vi "FPGA Wizard.vi"() -> ()   [LabVIEW 2015]
uses:
  Classes/Project/FPGA Settings.ctl
  Classes/Module/Module Class/Module Settings.ctl
  Classes/IO/IO Class/Signal Settings.ctl
  Classes/Project/Project.lvclass
  Classes/Loop/Block Diagram/Block Diagram.lvclass
  Classes/IO/IO Class/IO Class.lvclass
  Classes/Module/Module Class/Module.lvclass
panel:
  out "Array":T1[](array[typedef])
  out "error out":errorcluster
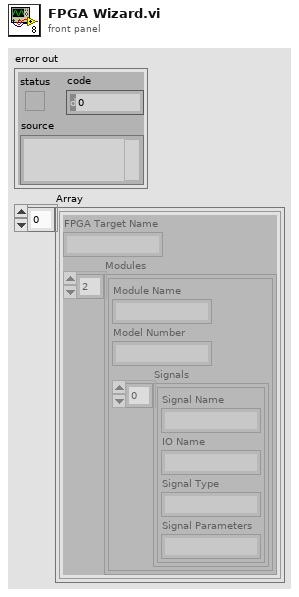
[diagram p1: front panel]
types:
  T1 = typedef "FPGA Settings.ctl" = cluster{"FPGA Target Name":string, "Modules":T2[]}
  T2 = typedef "Module.lvclass/Module Settings.ctl" = cluster{"Module Name":string, "Model Number":string, "Signals":T3[]}
  T3 = typedef "IO Class.lvclass/Signal Settings.ctl" = cluster{"Signal Name":string, "IO Name":string, "Signal Type":string, "Signal Parameters":string}
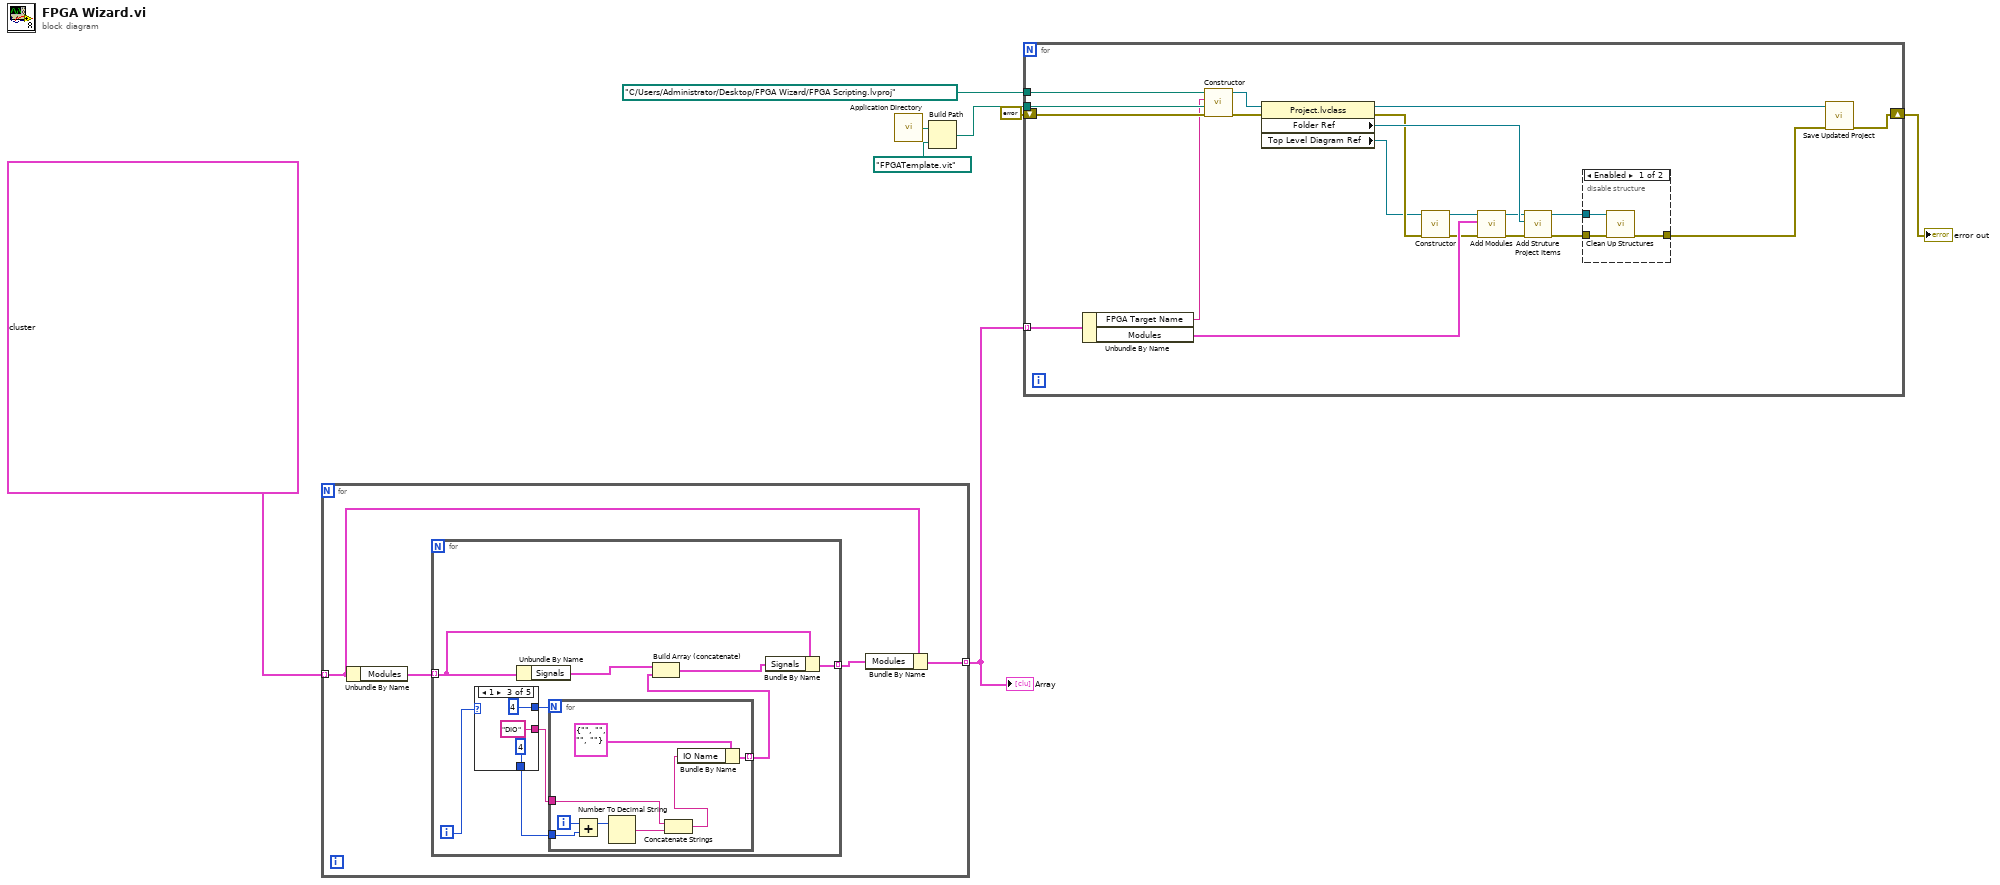
[diagram p0: block diagram]
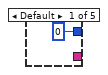
[diagram p2: hidden frame]
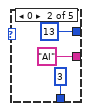
[diagram p3: hidden frame]
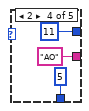
[diagram p4: hidden frame]
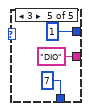
[diagram p5: hidden frame]
diagram:
  n1 = for {
    tunnel: T1[] [{"FPGA Target Name"="FPGA Target", "Modules"=[{"Module Name"="Mod1", "Model Number"="9220", "Signals"=[{"Signal Name"="Press", "IO Name"="AI0", "Signal Type"="Numeric Indicator", "Signal Parameters"=""}, {"Signal Name"="Temp", "IO Name"="AI1", "Signal Type"="Numeric Indicator", "Signal Parameters"=""}, {"Signal Name"="Injector", "IO Name"="AI2", "Signal Type"="Analog PWM Input", "Signal Parameters"=""}]}, {"Module Name"="Mod2", "Model Number"="9401", "Signals"=[{"Signal Name"="Relay State", "IO Name"="DIO0", "Signal Type"="Digital Indicator", "Signal Parameters"=""}, {"Signal Name"="Switch State", "IO Name"="DIO1", "Signal Type"="Digital Indicator", "Signal Parameters"=""}, {"Signal Name"="Key State", "IO Name"="DIO2", "Signal Type"="Digital Static Input", "Signal Parameters"=""}, {"Signal Name"="PWM State", "IO Name"="DIO3", "Signal Type"="Digital PWM Input", "Signal Parameters"=""}, {"Signal Name"="Cylinder 1 Injector", "IO Name"="DIO3", "Signal Type"="Digital Event", "Signal Parameters"="{\"Events\":4}"}]}, {"Module Name"="Mod3", "Model Number"="9264", "Signals"=[{"Signal Name"="Dyno Setpoint", "IO Name"="AO0", "Signal Type"="Numeric Control", "Signal Parameters"=""}, {"Signal Name"="Power Supply Setpoint", "IO Name"="AO1", "Signal Type"="Numeric Control", "Signal Parameters"=""}, {"Signal Name"="VR Sensor", "IO Name"="AO3", "Signal Type"="Analog Replay", "Signal Parameters"=""}, {"Signal Name"="Knock", "IO Name"="AO3", "Signal Type"="Knock Sensor", "Signal Parameters"="{\"Cyclinders\":6}"}, {"Signal Name"="Simple Knock", "IO Name"="AO4", "Signal Type"="Sine Output", "Signal Parameters"=""}]}, {"Module Name"="Mod4", "Model Number"="9401", "Signals"=[{"Signal Name"="Intake CAM", "IO Name"="DIO0", "Signal Type"="Digital Pattern", "Signal Parameters"=""}, {"Signal Name"="Exhaust CAM", "IO Name"="DIO1", "Signal Type"="Digital Pattern", "Signal Parameters"=""}, {"Signal Name"="Crank", "IO Name"="DIO2", "Signal Type"="Directional Sensor", "Signal Parameters"=""}, {"Signal Name"="Relay", "IO Name"="DIO3", "Signal Type"="Digital Control", "Signal Parameters"=""}, {"Signal Name"="Switch", "IO Name"="DIO4", "Signal Type"="Digital Control", "Signal Parameters"=""}, {"Signal Name"="PWM", "IO Name"="DIO5", "Signal Type"="Digital PWM Output", "Signal Parameters"=""}, {"Signal Name"="Key", "IO Name"="DIO6", "Signal Type"="Digital Static Output", "Signal Parameters"=""}]}, {"Module Name"="Mod5", "Model Number"="9401", "Signals"=[{"Signal Name"="Front Driver Wheel Speed", "IO Name"="DIO0, DIO1", "Signal Type"="Wheel Speed Sensor", "Signal Parameters"=""}, {"Signal Name"="Front Passenger Wheel Speed", "IO Name"="DIO2, DIO3", "Signal Type"="Wheel Speed Sensor", "Signal Parameters"=""}, {"Signal Name"="Rear Driver Wheel Speed", "IO Name"="DIO4, DIO5", "Signal Type"="Wheel Speed Sensor", "Signal Parameters"=""}, {"Signal Name"="Rear Passenger Wheel Speed", "IO Name"="DIO6,DIO7", "Signal Type"="Wheel Speed Sensor", "Signal Parameters"=""}]}]}] -> [w11] mode=indexing
    tunnel: [w9] -> w1 mode=indexing
    n2 = Unbundle By Name(w11) -> ("Modules"=w12:T2[])
    n3 = for {
      tunnel: w12 -> [w18] mode=indexing
      tunnel: [w16] -> w10 mode=indexing
      i -> [w15]
      n4 = case shown="1" w15 {
        tunnel: [0 13 4 11 1] -> w21
        tunnel: [_ "AI" "DIO" "AO" "DIO"] -> w14
        tunnel: [_ 3 ("y") 4 ("y") 5 ("y") 7 ("y")] -> w13
        frame Default {
        }
        frame 0 {
        }
        frame 1 {
        }
        frame 2 {
        }
        frame 3 {
        }
      }
      n5 = Unbundle By Name(w18) -> ("Signals"=w19:T3[])
      n6 = for {
        N: w21 -> [_]
        tunnel: [w37] -> w20 mode=indexing
        tunnel: w14 -> [w36]
        tunnel: w13 -> [w35]
        i -> [w42]
        n7 = Add(x=w42, y=w35) -> (x+y=w41:i32)
        n8 = Number To Decimal String(number=w41) -> (decimal integer string=w40:string)  [unwired: 1 in]
        n9 = Concatenate Strings(w36, w40) -> (w38:string)
        n10 = Bundle By Name(cluster=T3 {"Signal Name"="", "IO Name"="", "Signal Type"="", "Signal Parameters"=""}, "IO Name"=w38) -> (w37:T3)
      }
      n11 = Build Array (concatenate)(w19, w20) -> (w17:T3[])
      n12 = Bundle By Name(cluster=w18, "Signals"=w17) -> (w16:T2)
    }
    n13 = Bundle By Name(cluster=w11, "Modules"=w10) -> (w9:T1)
  }
  "Array" <- w1
  n14 = call <vilib>:"Application Directory.vi"() -> ("Application Directory"=w7:path)
  n15 = Build Path(base path=w7, name or relative path=path "FPGATemplate.vit" ("template")) -> (appended path=w5:path)
  n16 = for {
    tunnel: path "C:/Users/Administrator/Desktop/FPGA Wizard/FPGA Scripting.lvproj" ("Project Path") -> [w62]
    tunnel: w5 -> [w55]
    shift-right: [w46] -> w4
    shift-left: errorcluster {"status"=FALSE, "code"=0, "source"=""} ("error out") -> [w54]
    tunnel: w1 -> [w53] mode=indexing
    n17 = Unbundle By Name(w53) -> ("FPGA Target Name"=w52:string, "Modules"=w51:T2[])
    n18 = call "Constructor.vi"("error in (no error)"=w54, "FPGA Template Path"=w55, "FPGA Target Name"=w52, "Project Path"=w62) -> ("error out"=w60:errorcluster, "Project out"=w61:refnum<class "Project.lvclass">)  [unwired: 6 in]
    n19 = property class="Project.lvclass"(reference=w61, error in=w60) -> (reference out=w56:refnum<class "Project.lvclass">, error out=w58:errorcluster, "Folder Ref"=w59:refnum<vi>, "Top Level Diagram Ref"=w57:refnum<vi>)
    n20 = call "Constructor.vi"("error in (no error)"=w58, "Top Level Diagram"=w57) -> ("error out"=w48:errorcluster, "Block Diagram"=w47:refnum<class "Block Diagram.lvclass">)  [unwired: 8 in]
    n21 = call "Add Modules.vi"("error in (no error)"=w48, "Modules"=w51, "Block Diagram in"=w47) -> ("error out"=w49:errorcluster, "Block Diagram out"=w50:refnum<class "Block Diagram.lvclass">)  [unwired: 7 in]
    n22 = call "Add Struture Project Items.vi"("error in (no error)"=w49, "Folder Location Ref"=w59, "Block Diagram in"=w50) -> ("error out"=w45:errorcluster, "Block Diagram out"=w43:refnum<class "Block Diagram.lvclass">)  [unwired: 7 in]
    n23 = disable-structure shown="Enabled" {
      disable-tunnel: w45 -> [w65 w66]
      disable-tunnel: [w64 w66] -> w44
      disable-tunnel: w43 -> [w63 _]
      frame Enabled {
        n24 = call "Clean Up Structures.vi"("error in (no error)"=w65, "Block Diagram in"=w63) -> ("error out"=w64:errorcluster)  [unwired: 8 in, 1 out]
      }
      frame Disabled {
      }
    }
    n25 = call-dynamic "Save Updated Project.vi"("error in (no error)"=w44, "Project in"=w56) -> ("error out"=w46:errorcluster)  [unwired: 8 in, 1 out]
  }
  "error out" <- w4
